vi "Set Bucket.vi"(8 "error in (no error)":errorcluster, 10 "Bucket name":string, 11 "Data.S3 2":refnum<class "Data.S3.lvclass">) -> (0 "error out":errorcluster, 3 "Data.S3":refnum<class "Data.S3.lvclass">)   [LabVIEW 2020, in "Data.S3.lvclass"]
uses:
  Data.S3.lvclass
  Data.S3.lvclass/Data.S3.ctl
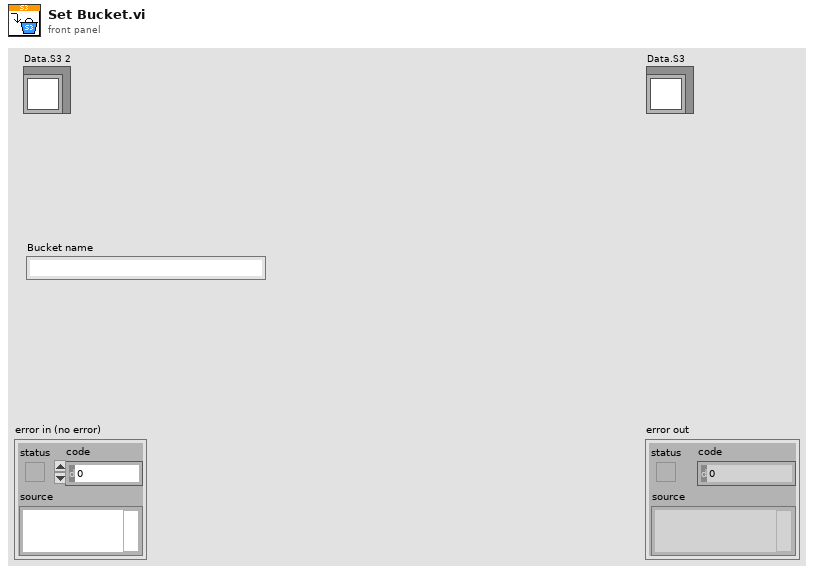
[diagram p1: front panel]
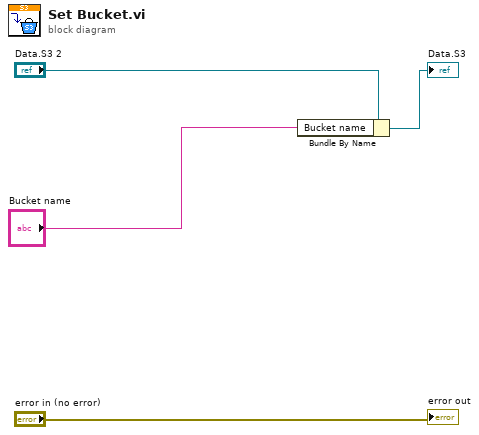
[diagram p0: block diagram]
diagram:
  n1 = Bundle By Name(cluster="Data.S3 2", "Bucket name"="Bucket name") -> (→"Data.S3":refnum<class "Data.S3.lvclass">)
  "error out" <- "error in (no error)"
